vi "sub_single-cycle-cnt.vi"(11 "Single sequence":T1 {"Ch" min=1 max=6 step=1}) -> ()   [LabVIEW 2019]
uses:
  sequence_single.ctl
  _ctrl/Sinple-sequence-type.ctl
  _ctrl/rw.ctl
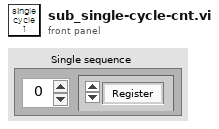
[diagram p1: front panel]
types:
  T1 = typedef "sequence_single.ctl" = cluster{"Type":T2, "Ch":u16}
  T2 = typedef "Sinple-sequence-type.ctl" = enum16{"Register", "RC", "B1", "B2", "B3"}
  T3 = typedef "rw.ctl" = enum16{"read", "write"}
  T4 = cluster{"DL950_config":refnum<vi>, "BP4610 Config":refnum<vi>, "DSP1950 Config":refnum<vi>, "2470-config":refnum<vi>, "cDAQ 9269 AO config":refnum<vi>, "cDAQ 9221 Config":refnum<vi>, "cDAQ-9467 Config":refnum<vi>, "Waveform":refnum<vi>, "DL950 wfm":refnum<vi>, "AI Graph":refnum<vi>, "AO_Wave-config":refnum<vi>, "DL950 items":refnum<vi>, "Volt":refnum<vi>, "Current":refnum<vi>, "AO_Level":refnum<vi>, "RCconfig":refnum<vi>}
  T5 = typedef "cap_config.ctl" = cluster{"제어 전압[V]":dbl, "출력전압[V]":dbl, "전류[A]":dbl, "출력전류[A]":dbl, "ON[초]":dbl, "OFF[초]":dbl, "시험횟수[N]":u32, "방전 진단[V]":dbl, "전압98[초]":dbl, "전압63[초]":dbl, "전류37[초]":dbl, "방전 시간[초]":dbl, "전압98[+/-%]":dbl, "전압63[+/-%]":dbl, "전류37[+/-%]":dbl, "Ch selection":cluster{"ch 1":bool, "ch 2":bool, "ch 3":bool, "ch 4":bool, "ch 5":bool, "ch 6":bool}, "사이클[N]":u32}
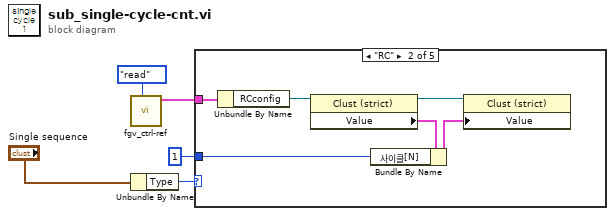
[diagram p0: block diagram]
diagram:
  n1 = call "fgv_ctrl-ref.vi"("cmd"=rw."read") -> ("output cluster 2"=w2:T4)  [unwired: 9 in, 1 out]
  n2 = Unbundle By Name("Single sequence") -> ("Type"=w5:T2)
  n3 = case shown="\"RC\"" w5 {
    tunnel: w2 -> [_ w11 _ _ _]
    tunnel: u32 1 ("사이클[N]") -> [_ w8 _ _ _]
    frame "Register", Default {
    }
    frame "RC" {
      n4 = Unbundle By Name(w11) -> ("RCconfig"=w10:refnum<vi>)
      n5 = property class="Clust (strict)"(reference=w10) -> (reference out=w7:refnum<vi>, "Value"=w9:T5)  [unwired: 1 in, 1 out]
      n6 = Bundle By Name(cluster=w9, "사이클[N]"=w8) -> (w6:T5)
      n7 = property class="Clust (strict)"(reference=w7, "Value"=w6) -> ()  [unwired: 1 in, 2 out]
    }
    frame "B1" {
    }
    frame "B2" {
    }
    frame "B3" {
    }
  }
